vi "CalcData.vi"(8 "error in (no error)":errorcluster, 10 "Complex Data (in)":csg[](array[numeric])) -> (0 "error out":errorcluster, 2 "Array out":csg[](array[numeric]))   [LabVIEW 2014]
uses:
  GlobalVariables.vi
  <vilib>/Utility/error.llb/Error Cluster From Error Code.vi
  <vilib>/rvi/errors/niLvFpgaAdjustHostInterfaceError.vi
  <vilib>/rvi/interface/nirviMethod/nirviMethod.xnode
  <vilib>/rvi/errors/niLvFpgaMergeErrorWithErrorCode.vi
  <vilib>/FPGAPlugInAG/Dynamic/niLvFpga_ReadFifo_Dynamic.vi
  <vilib>/FPGAPlugInAG/Dynamic/niLvFpga_WriteFifo_Dynamic.vi
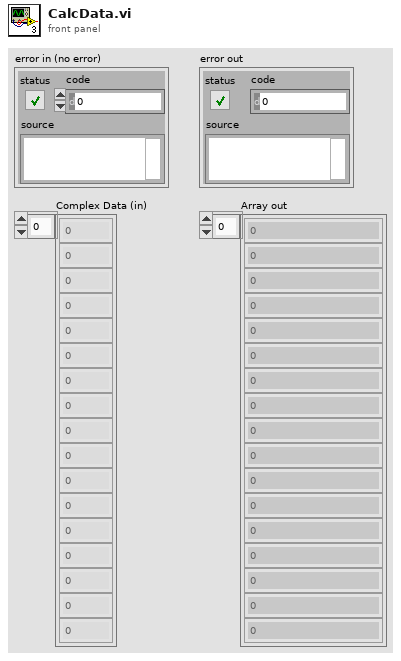
[diagram p1: front panel]
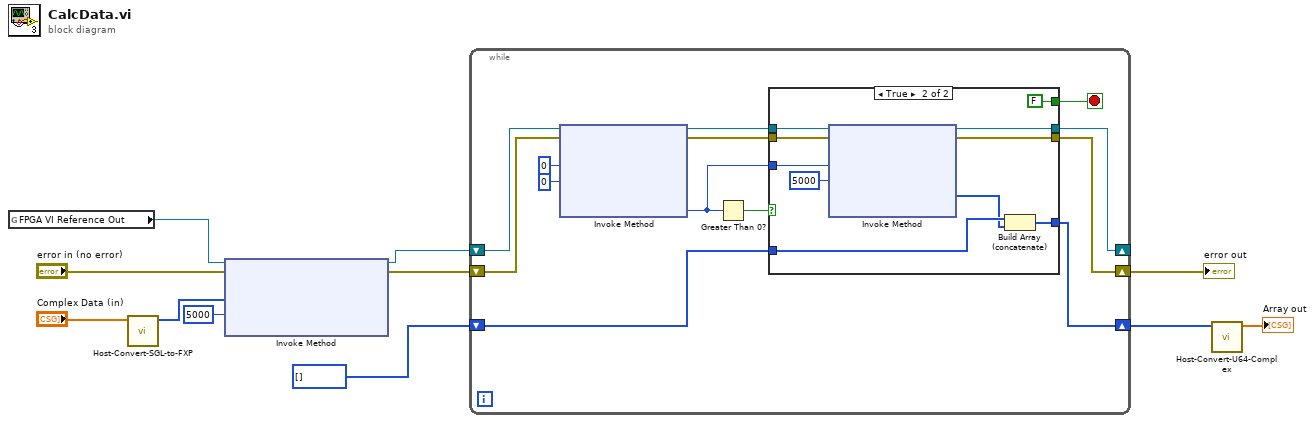
[diagram p0: block diagram]
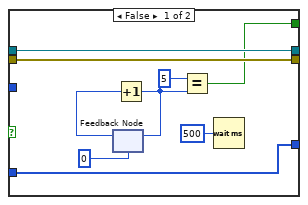
[diagram p2: hidden frame]
diagram:
  n1 = global read "GlobalVariables.vi" "FPGA VI Reference Out"() -> (w1:refnum<k20>)
  n2 = call "Host-Convert-SGL-to-FXP.vi"("Complex Data (in)"="Complex Data (in)") -> ("Complex Data Ready for FPGA (out)"=w11:u64[])  [unwired: 10 in]
  n3 = xnode "Invoke Method"("FPGA VI Reference In"=w1, "error in"="error in (no error)", "Data"=w11, "Timeout (ms)"=5000) -> ("FPGA VI Reference Out"=w4:refnum<k20>, "error out"=w5:errorcluster)  [unwired: 1 out]
  n4 = while {
    shift-right: [w13] -> _
    shift-left: w4 -> [w24]
    shift-right: [w14] -> w6
    shift-left: w5 -> [w15]
    shift-right: [w18] -> w9
    shift-left: u64[] [] -> [w17]
    stop <- w12 stop-if-true
    n5 = xnode "Invoke Method"("FPGA VI Reference In"=w24, "error in"=w15, "Number of Elements"=u32 0, "Timeout (ms)"=0) -> ("FPGA VI Reference Out"=w20:refnum<k20>, "error out"=w16:errorcluster, "Elements Remaining"=w19:u32)  [unwired: 1 out]
    n6 = Greater Than 0?(x=w19) -> (x > 0?=w21:bool)
    n7 = case shown="True" w21 {
      tunnel: w20 -> [w31 w43]
      tunnel: w19 -> [_ w42]
      tunnel: [w33 w38] -> w18
      tunnel: w17 -> [w33 w40]
      tunnel: w16 -> [w32 w37]
      tunnel: [w32 w36] -> w14
      tunnel: [w31 w35] -> w13
      tunnel: [w26 FALSE] -> w12
      frame False {
        n8 = feedback #1(0) -> (w29:i32)
        n9 = Increment(x=w29) -> (x+1=w28:i32)
        n10 = feedback-in #1(w28) -> ()
        n11 = Equal?(x=5, y=w28) -> (x = y?=w26:bool)
        n12 = Wait (ms)(milliseconds to wait=u32 500) -> ()  [unwired: 1 out]
      }
      frame True {
        n13 = xnode "Invoke Method"("FPGA VI Reference In"=w43, "error in"=w37, "Number of Elements"=w42, "Timeout (ms)"=5000) -> ("FPGA VI Reference Out"=w35:refnum<k20>, "error out"=w36:errorcluster, "Data"=w39:u64[])  [unwired: 1 out]
        n14 = Build Array (concatenate)(w40, w39) -> (w38:u64[])
      }
    }
  }
  "error out" <- w6
  n15 = call "Host-Convert-U64-Complex.vi"("Array in"=w9) -> ("Array out"=→"Array out":csg[])  [unwired: 10 in]
